vi "GDX_NoPopups.vi"() -> ()   [LabVIEW 2019]
panel:
  in  "Channel On/Off Array":bool[](array[boolean])=[TRUE, FALSE, FALSE, FALSE, FALSE, FALSE, FALSE, FALSE, FALSE, FALSE, FALSE, FALSE]
  in  "Device Name Array":string[](array[string])
  in  "Sample Rate (samples/sec)":dbl=10.0
  out "XY Graph":cluster{dbl[], dbl[]}[](graph)
  in  "stop":bool
  # "If you run the other examples, like Chart, Meter or XYGraph, you will notice that connecting the GDX sensor, choosing the channels, and setting the sample rate are all done with popup dialog boxes. You do not have to use these dialog boxes. You can also hardcode in the device, the sample rate and the channels in the block diagram, or use front panel controls, like this example."
  # "You can connect your GDX device without using the popup dialog. The \"Name\" is the device's order code followed by the device's serial number (with a space in-between).  The serial number can be found on the device. Examples of what the name would look like are:\nGDX-FOR 071000U9\nGDX-ACC 0H1017F0\nGDX-LC 091000C3\nIn this example you only enter a single device name. Enter your device's name in the first element of the array control above before running this program. Note that if you create an example that uses several GDX sensors then you would simply put the other names as the next elements in the Device Name Array control."
  # "If you know what channels you want to read when you run your program, you can use the On/Off array to input which channels are active. Run the GetSensorInfo example VI if you want to see how many channels your GDX device has. Note that not all channels will be in order. For example, the Light and Color sensor has 5 channels. Ch 1 is light, Ch 2 is UV, and Channels 5,6 and 7 are color. There are no Channels 3 or 4, so your On/Off array would be On, On, Off, Off, On, On, On."
  # "To avoid the sample rate popup dialog, simply send the sample rate to the program using this control (or hardcoded on the block diagram)."
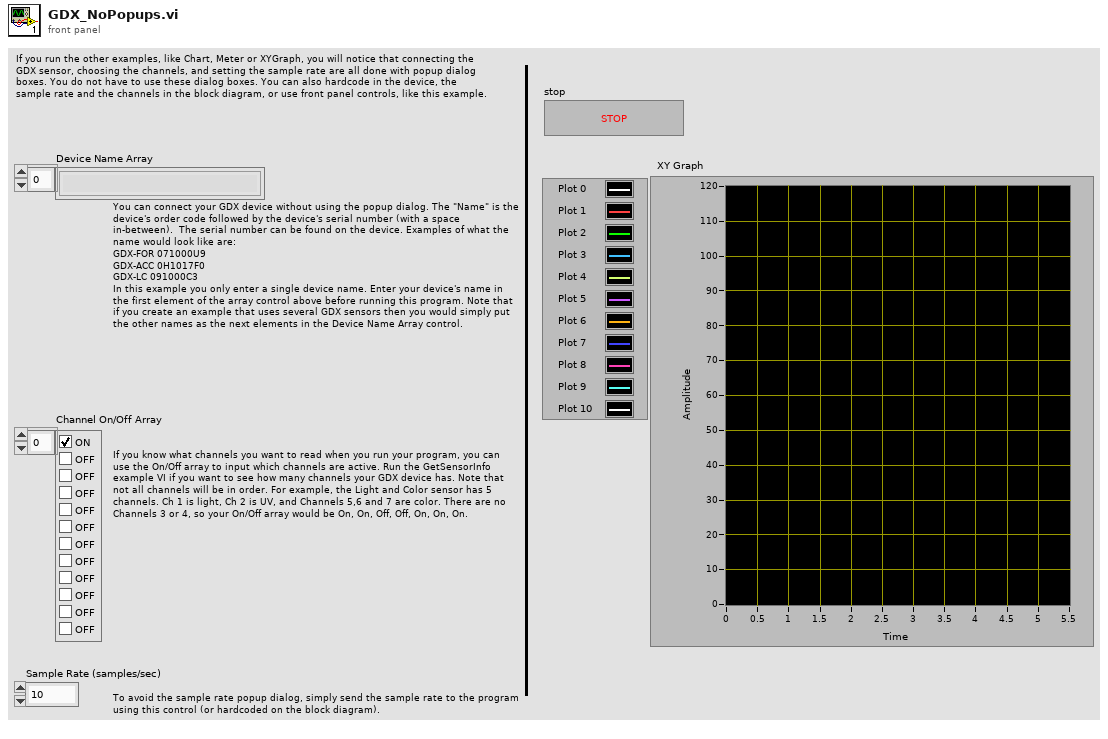
[diagram p1: front panel]
types:
  T1 = enum16{"Open from Dialog Popup", "Open all Available Devices", "Input Device Names"}
  T2 = enum16{"Activate from Dialog Popup", "Activate All Channels", "Input On/Off Array", "Input Channel  Mask", "Burn Sensor Default Channels"}
  T3 = enum16{"Set Rate from Dialog Popup", "Default 1 Sample/Sec", "Input Sample Rate"}
  T4 = typedef "D2PIO_D2PIOCluster.ctl" = cluster{"Library Handle":i64, "Device List Handle":i64, "BT Device Handles":i64[], "USB Device Handles":i64[], "BT+USB Device Handles":i64[], "Measurement Tick":dbl[], "Ch Availability Mask":u32[]}
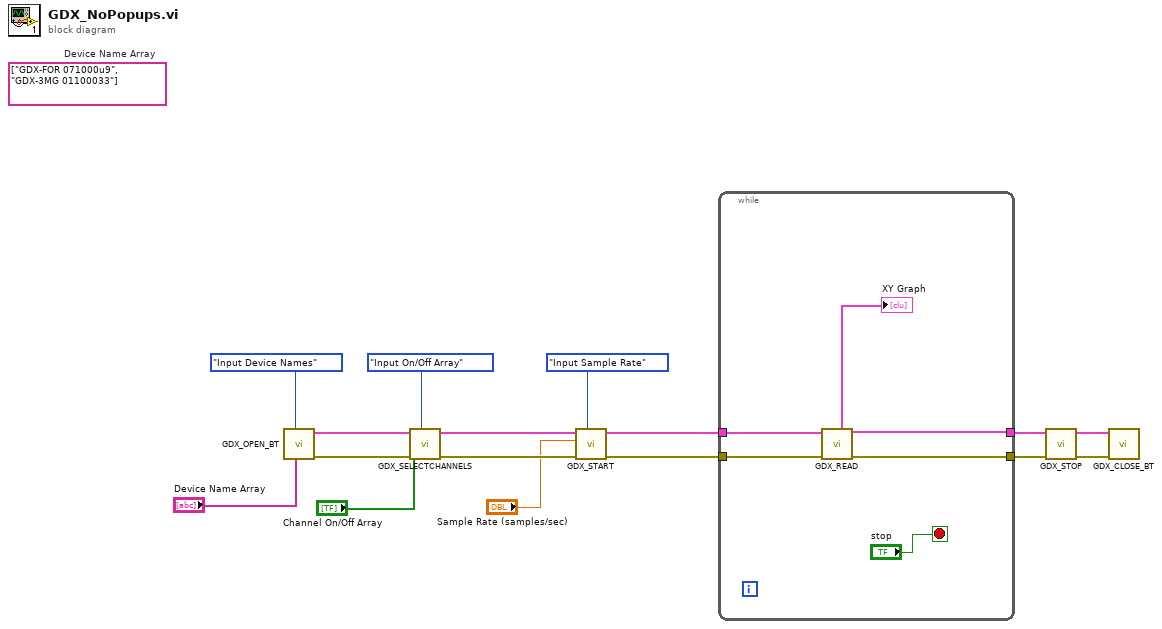
[diagram p0: block diagram]
diagram:
  (unwired) string[] ["GDX-FOR 071000u9", "GDX-3MG 01100033"]  # Device Name Array
  n1 = call <vilib>:"GDX_OPEN_BT.vi"("Device Name Array"="Device Name Array", "Enum"=T1."Input Device Names") -> ("error out"=w10:errorcluster, "D2PIO Cluster Out"=w11:T4)  [unwired: 8 in]
  n2 = call <vilib>:"GDX_SELECTCHANNELS.vi"("Enum"=T2."Input On/Off Array", "error in (no error)"=w10, "Channel On/Off Array"="Channel On/Off Array", "D2PIO Cluster In"=w11) -> ("error out"=w7:errorcluster, "D2PIO Cluster Out"=w8:T4)  [unwired: 6 in]
  n3 = call <vilib>:"GDX_START.vi"("Enum"=T3."Input Sample Rate", "error in (no error)"=w7, "Sample Rate (samples/sec)"="Sample Rate (samples/sec)", "D2PIO Cluster In"=w8) -> ("error out"=w16:errorcluster, "D2PIO Cluster Out"=w15:T4)  [unwired: 4 in, 2 out]
  n4 = while {
    tunnel: w16 -> [w22]
    tunnel: w15 -> [w20]
    tunnel: [w17] -> w14
    tunnel: [w18] -> w9
    stop <- "stop" stop-if-true
    n5 = call <vilib>:"GDX_READ.vi"("error in (no error)"=w22, "D2PIO Cluster In"=w20) -> ("error out"=w18:errorcluster, "D2PIO Cluster Out"=w17:T4, "XY Graph Data"=→"XY Graph":cluster{dbl[], dbl[]}[])  [unwired: 4 in, 3 out]
  }
  n6 = call <vilib>:"GDX_STOP.vi"("error in (no error)"=w9, "D2PIO Cluster In"=w14) -> ("error out"=w12:errorcluster, "D2PIO Cluster Out"=w13:T4)  [unwired: 8 in]
  n7 = call <vilib>:"GDX_CLOSE_BT.vi"("error in (no error)"=w12, "D2PIO Cluster In"=w13) -> ()  [unwired: 8 in, 2 out]
